vi "FM_IQ_Filter.vi"(2 "Sample freq":dbl, 7 "Array in":cdb[](array[numeric])) -> (8 "Array":cdb[](array[numeric]))   [LabVIEW 2020]
uses:
  <vilib>/Analysis/3filter.llb/Elliptic Filter (DBL).vi
  <vilib>/Analysis/NI_AALBase.lvlib
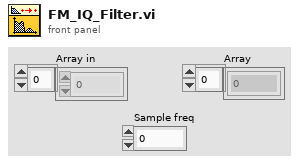
[diagram p1: front panel]
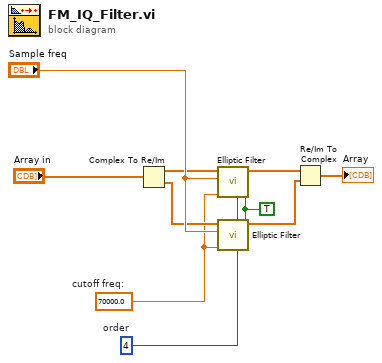
[diagram p0: block diagram]
diagram:
  w1 = 70000.0  # cutoff freq:
  w6 = TRUE ("init/cont (init:F)")
  w7 = 4  # order
  n1 = Complex To Re/Im(x + iy="Array in") -> (x=w5:dbl[], y=w4:dbl[])
  n2 = call-poly <vilib>:"Elliptic Filter.vi"("init/cont (init:F)"=w6, "order"=w7, "low cutoff freq: fl"=w1, "sampling freq: fs"="Sample freq", "X"=w5) -> ("Filtered X"=w2:dbl[])  [unwired: 5 in, 1 out]
  n3 = call-poly <vilib>:"Elliptic Filter.vi"("init/cont (init:F)"=w6, "order"=w7, "low cutoff freq: fl"=w1, "sampling freq: fs"="Sample freq", "X"=w4) -> ("Filtered X"=w3:dbl[])  [unwired: 5 in, 1 out]
  n4 = Re/Im To Complex(1:w3, 2:w2) -> (0:→"Array":cdb[])
